vi "Pointer Convert TDMS V3.vi"() -> ()   [LabVIEW 2014]
doc: "Reads a TDMS (Technical Data Management Streaming) file."
panel:
  in  "Tab Control":enum32{"Control", "Help"}(tab)
  in  "Input path:":path
  out "Output path:":path
  out "Number of converted files:":i32
  out "Version":string
  out "array of strings":string[](array[string])
  out "channel names":string[](array[string])
  out "error out":errorcluster
  in  "error in (no error) 3":errorcluster
  in  "error in (no error) 2":errorcluster
  out "channel names 2":string[](array[string])
  out "array of strings 2":string[](array[string])
  # "Please select the folder or file you want to convert here:"
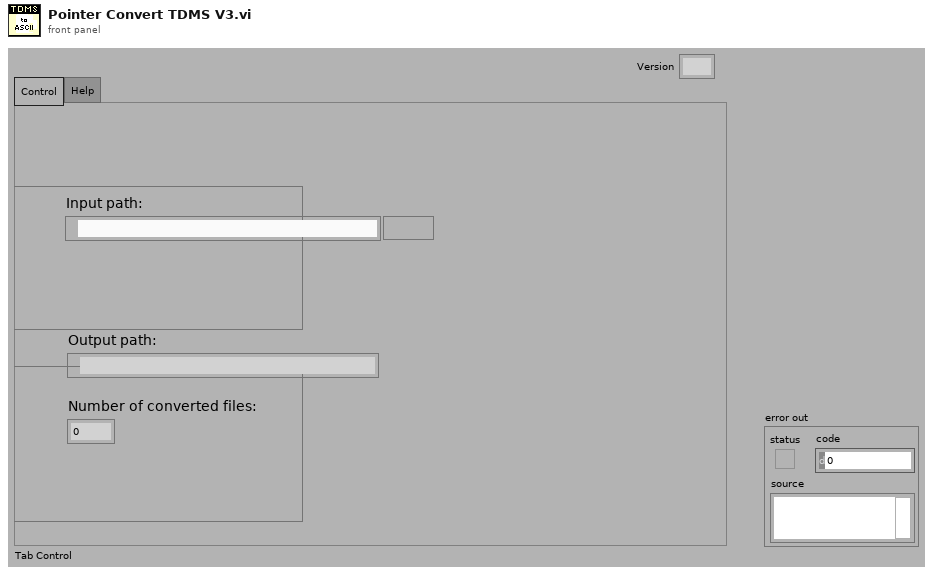
[diagram p1: front panel]
types:
  T1 = enum16{"open", "replace", "create", "open or create", "replace or create", "replace or create with confirmation"}
  T2 = enum16{"open", "open or create", "create or replace", "create", "open (read-only)"}
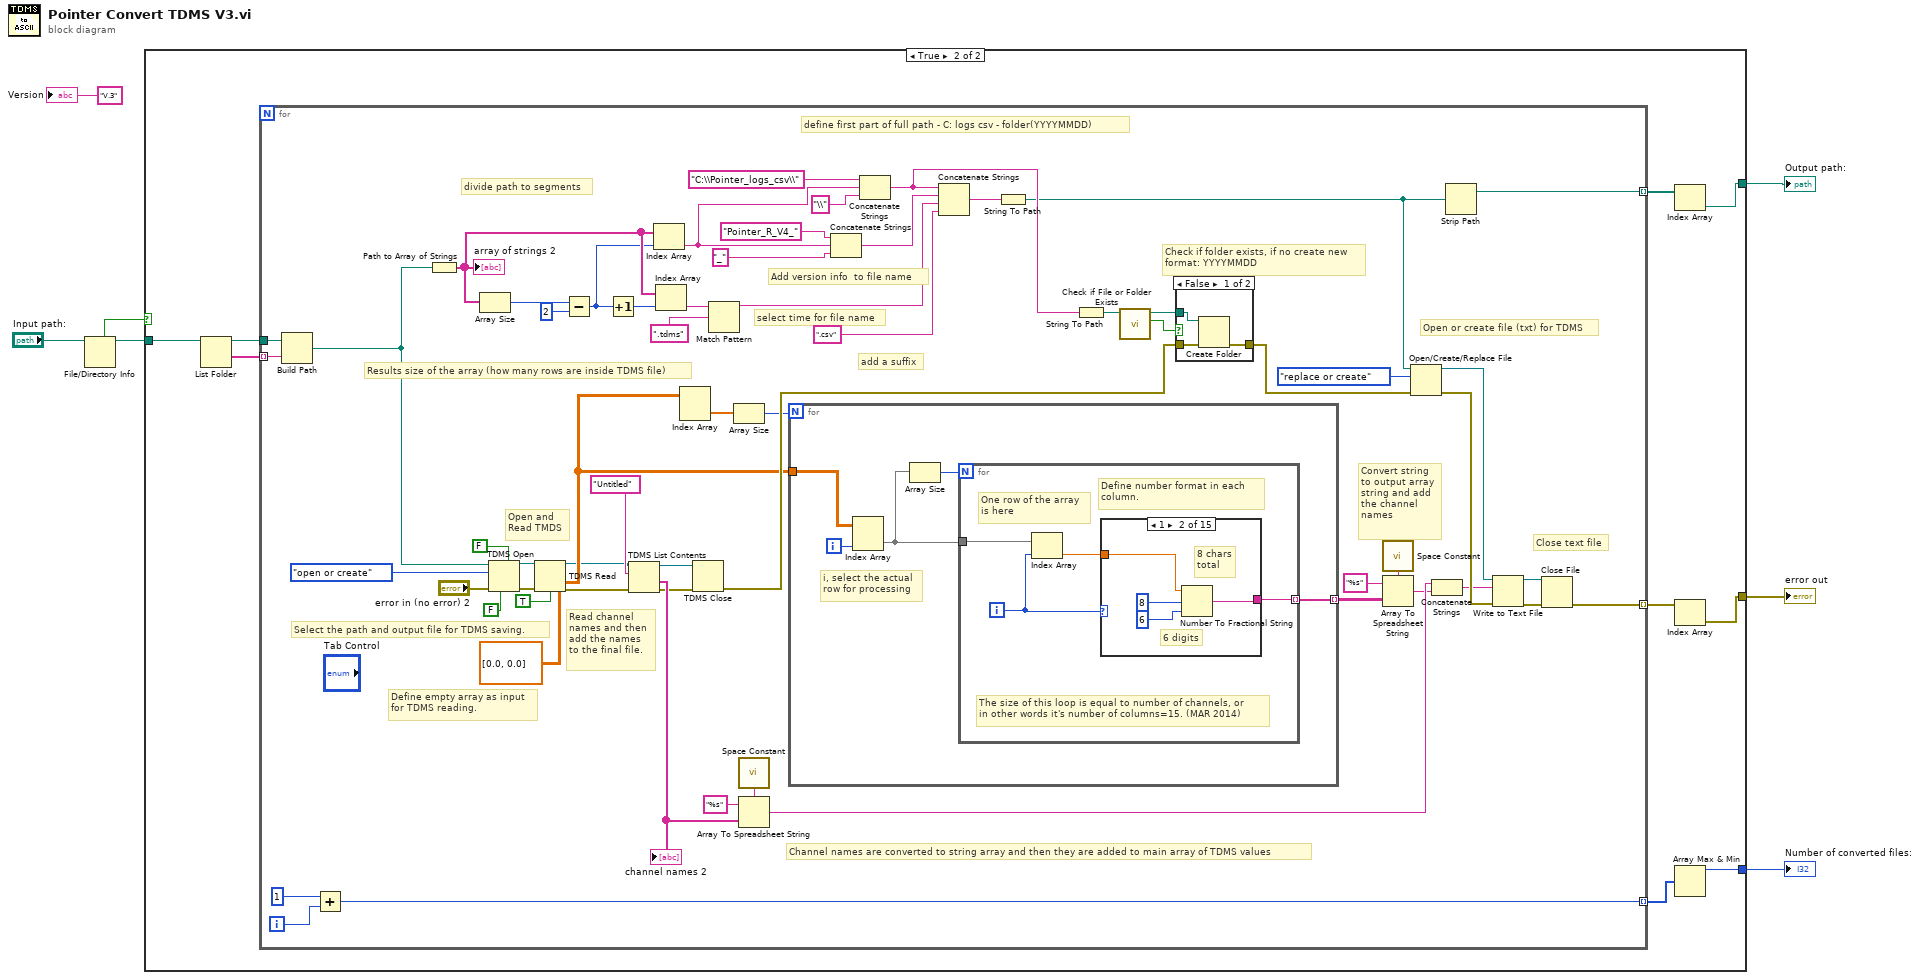
[diagram p0: block diagram]
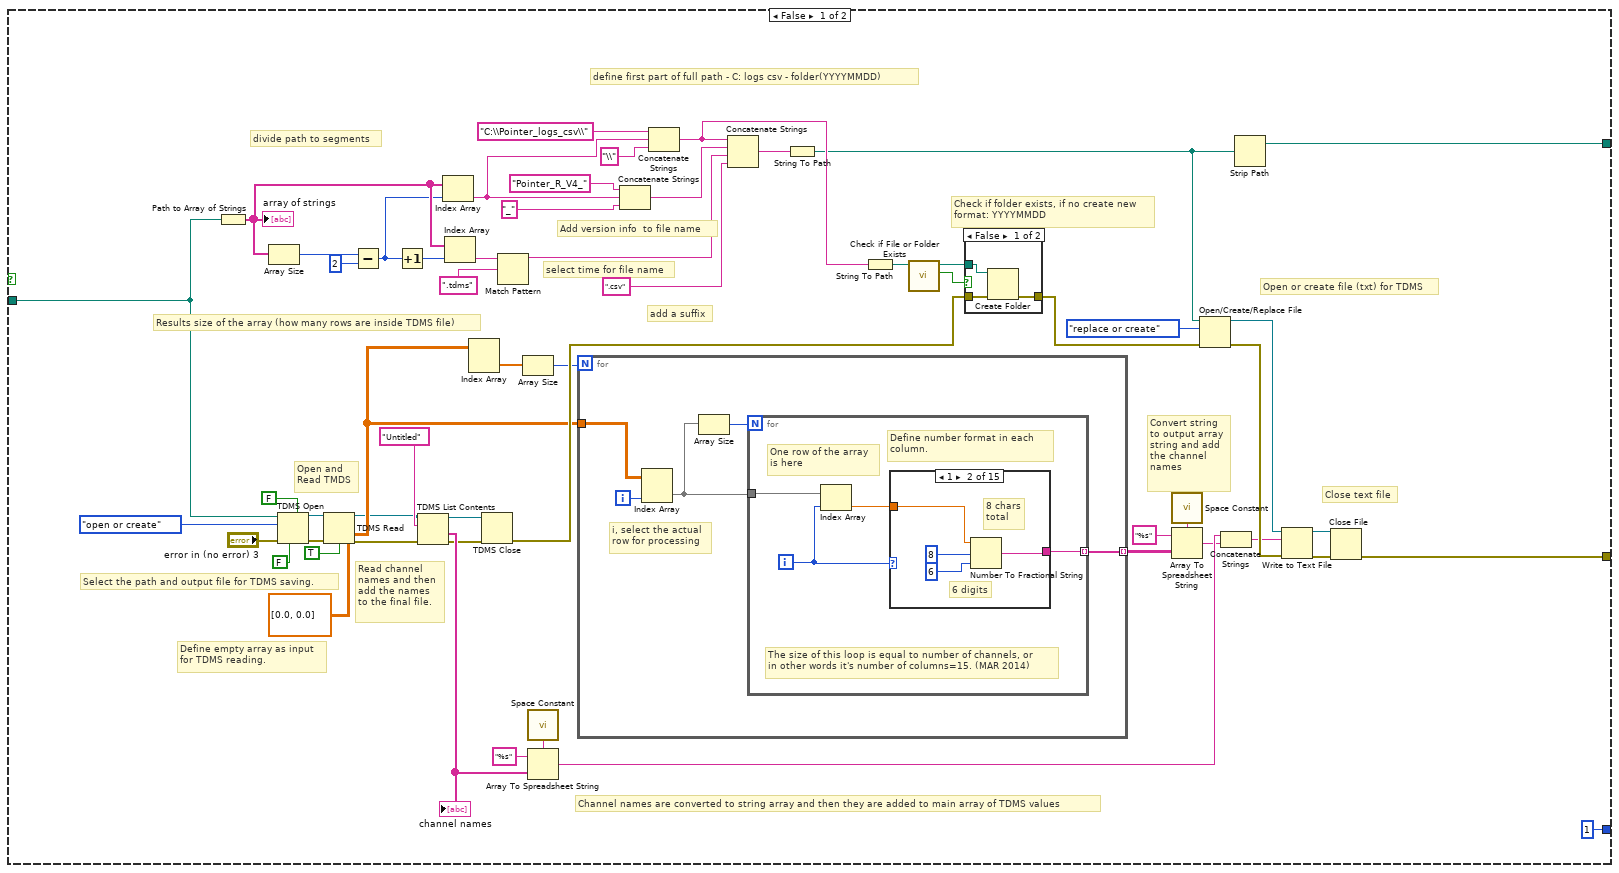
[diagram p2: hidden frame]
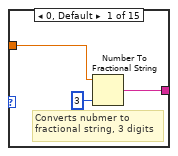
[diagram p4: hidden frame]
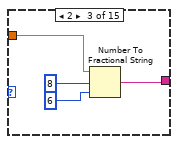
[diagram p5: hidden frame]
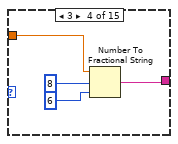
[diagram p6: hidden frame]
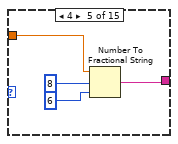
[diagram p7: hidden frame]
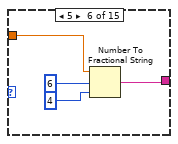
[diagram p8: hidden frame]
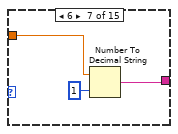
[diagram p9: hidden frame]
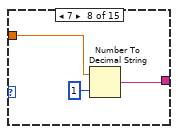
[diagram p10: hidden frame]
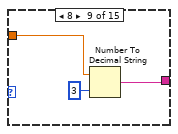
[diagram p11: hidden frame]
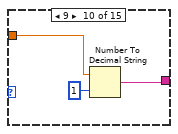
[diagram p12: hidden frame]
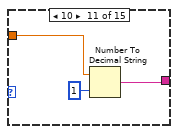
[diagram p13: hidden frame]
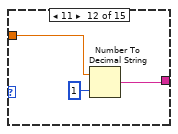
[diagram p14: hidden frame]
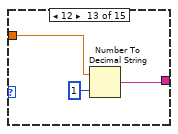
[diagram p15: hidden frame]
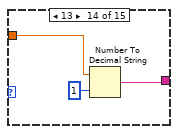
[diagram p16: hidden frame]
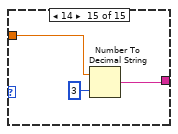
[diagram p17: hidden frame]
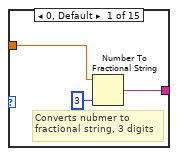
[diagram p19: hidden frame]
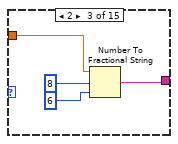
[diagram p20: hidden frame]
diagram:
  n1 = File/Directory Info(path="Input path:") -> (path out=w5:path, directory=w6:bool)  [unwired: 1 in, 5 out]
  n2 = case shown="True" w6 {
    tunnel: w5 -> [w11 w134]
    tunnel: [w10 w132] -> w4
    tunnel: [w9 w130] -> w3
    tunnel: [1 w128] -> w2
    frame False {
      # "add a suffix"
      # "select time for file name"
      # "Add version info  to file name"
      # "Check if folder exists, if no create new\nformat: YYYYMMDD"
      # "define first part of full path - C: logs csv - folder(YYYYMMDD)"
      # "divide path to segments"
      # "Open or create file (txt) for TDMS"
      # "Convert string\nto output array\nstring and add \nthe channel \nnames"
      # "Close text file"
      # "Channel names are converted to string array and then they are added to main array of TDMS values"
      # "Define empty array as input\nfor TDMS reading."
      # "Results size of the array (how many rows are inside TDMS file)"
      # "Open and \nRead TMDS"
      # "Read channel\nnames and then\nadd the names \nto the final file."
      # "Select the path and output file for TDMS saving."
      n3 = Path to Array of Strings(0:w11) -> (2:w45:string[])  [unwired: 1 out]
      "array of strings" <- w45
      n4 = Array Size(array=w45) -> (size(s)=w41:i32)
      n5 = TDMS Open(5:FALSE ("create index file? (T)"), 6:FALSE ("disable buffering (T)"), 8:"error in (no error) 3", 10:T2."open or create" ("operation"), 11:w11) -> (0:w15:errorcluster, 3:w14:refnum<k34>)  [unwired: 2 in]
      n6 = TDMS Read(0:w14, 11:w15, 12:dbl[][] [[0.0, 0.0]], 13:TRUE ("return channels in file order? (F)")) -> (4:w20:refnum<k34>, 10:w29:dbl[][], 15:w23:errorcluster)  [unwired: 4 in, 3 out]
      n7 = Subtract(x=w41, y=2) -> (x-y=w43:i32)
      n8 = Increment(x=w43) -> (x+1=w44:i32)
      n9 = TDMS List Contents(4:w23, 6:"Untitled" ("group name"), 7:w20) -> (0:w24:errorcluster, 1:w32:string[], 3:w21:refnum<k34>)  [unwired: 1 out]
      "channel names" <- w32
      n10 = Index Array(array=w45, index=w43) -> (element=w56:string)
      n11 = Index Array(array=w45, index=w44) -> (element=w47:string)
      n12 = Index Array(array=w29) -> (element=w27:dbl[])  [unwired: 2 in]
      n13 = TDMS Close(8:w24, 11:w21) -> (0:w57:errorcluster)  [unwired: 1 out]
      n14 = Match Pattern(string=w47, regular expression=".tdms") -> (before substring=w51:string)  [unwired: 1 in, 3 out]
      n15 = Array Size(array=w27) -> (size(s)=w28:i32)
      n16 = call <vilib>:"Space Constant.vi"() -> ("String"=w33:string)
      n17 = Array To Spreadsheet String(delimiter (Tab)=w33, array=w32, 3:"%s" ("format string")) -> (spreadsheet string=w37:string)
      n18 = for {
        N: w28 -> [_]
        tunnel: w29 -> [w73]
        tunnel: [w69] -> w35 mode=indexing
        i -> [w70]
        # "i, select the actual\nrow for processing"
        n19 = Index Array(array=w73, index (col)=w70) -> (element=w72:dbl[])  [unwired: 1 in]
        n20 = Array Size(array=w72) -> (size(s)=w71:i32)
        n21 = for {
          N: w71 -> [_]
          tunnel: w72 -> [w77]
          tunnel: [w75] -> w69 mode=indexing
          i -> [w74]
          # "One row of the array\nis here"
          # "Define number format in each \ncolumn."
          # "The size of this loop is equal to number of channels, or\nin other words it's number of columns=15. (MAR 2014)"
          n22 = Index Array(array=w77, index=w74) -> (element=w76:dbl)
          n23 = case shown="1" w74 {
            tunnel: w76 -> [w80 w82 w86 w90 w94 w98 w102 w105 w108 w111 w114 w117 w120 w123 w126]
            tunnel: [w79 w83 w87 w91 w95 w99 w103 w106 w109 w112 w115 w118 w121 w124 w127] -> w75
            frame 0, Default {
              # "Converts nubmer to \nfractional string, 3 digits"
              n24 = Number To Fractional String(number=w80, precision (6)=i16 3) -> (F-format string=w79:string)  [unwired: 2 in]
            }
            frame 1 {
              # "6 digits"
              # "8 chars\ntotal"
              n25 = Number To Fractional String(number=w82, width (-)=i16 8, precision (6)=i16 6) -> (F-format string=w83:string)  [unwired: 1 in]
            }
            frame 2 {
              n26 = Number To Fractional String(number=w86, width (-)=i16 8, precision (6)=i16 6) -> (F-format string=w87:string)  [unwired: 1 in]
            }
            frame 3 {
              n27 = Number To Fractional String(number=w90, width (-)=i16 8, precision (6)=i16 6) -> (F-format string=w91:string)  [unwired: 1 in]
            }
            frame 4 {
              n28 = Number To Fractional String(number=w94, width (-)=i16 8, precision (6)=i16 6) -> (F-format string=w95:string)  [unwired: 1 in]
            }
            frame 5 {
              n29 = Number To Fractional String(number=w98, width (-)=i16 6, precision (6)=i16 4) -> (F-format string=w99:string)  [unwired: 1 in]
            }
            frame 6 {
              n30 = Number To Decimal String(number=w102, width (-)=i16 1) -> (decimal integer string=w103:string)
            }
            frame 7 {
              n31 = Number To Decimal String(number=w105, width (-)=i16 1) -> (decimal integer string=w106:string)
            }
            frame 8 {
              n32 = Number To Decimal String(number=w108, width (-)=i16 3) -> (decimal integer string=w109:string)
            }
            frame 9 {
              n33 = Number To Decimal String(number=w111, width (-)=i16 1) -> (decimal integer string=w112:string)
            }
            frame 10 {
              n34 = Number To Decimal String(number=w114, width (-)=i16 1) -> (decimal integer string=w115:string)
            }
            frame 11 {
              n35 = Number To Decimal String(number=w117, width (-)=i16 1) -> (decimal integer string=w118:string)
            }
            frame 12 {
              n36 = Number To Decimal String(number=w120, width (-)=i16 1) -> (decimal integer string=w121:string)
            }
            frame 13 {
              n37 = Number To Decimal String(number=w123, width (-)=i16 1) -> (decimal integer string=w124:string)
            }
            frame 14 {
              n38 = Number To Decimal String(number=w126, width (-)=i16 3) -> (decimal integer string=w127:string)
            }
          }
        }
      }
      n39 = Concatenate Strings("Pointer_R_V4_" ("string"), w56, "_" ("string")) -> (w50:string)
      n40 = Concatenate Strings("C:\\Pointer_logs_csv\\", w56, "\\") -> (w59:string)
      n41 = Concatenate Strings(w59, w50, w51, ".csv" ("string")) -> (w52:string)
      n42 = String To Path(string=w52) -> (path=w12:path)
      n43 = String To Path(string=w59) -> (path=w60:path)
      n44 = call <vilib>:"Check if File or Folder Exists.vi"("path"=w60) -> ("file or folder exists?"=w61:bool, "dup path"=w62:path)  [unwired: 8 in, 1 out]
      n45 = case shown="False" w61 {
        tunnel: w57 -> [w67 w68]
        tunnel: [w66 w68] -> w58
        tunnel: w62 -> [w65 _]
        frame False {
          n46 = Create Folder(path (use dialog)=w65, error in=w67) -> (error out=w66:errorcluster)  [unwired: 1 in, 2 out]
        }
        frame True {
        }
      }
      n47 = call <vilib>:"Space Constant.vi"() -> ("String"=w31:string)
      n48 = Array To Spreadsheet String(delimiter (Tab)=w31, array=w35, 3:"%s" ("format string")) -> (spreadsheet string=w36:string)
      n49 = Open/Create/Replace File(file path (use dialog)=w12, error in=w58, operation (0:open)=T1."replace or create") -> (refnum out=w39:refnum<file>, error out=w40:errorcluster)  [unwired: 3 in, 1 out]
      n50 = Concatenate Strings(w37, w36) -> (w38:string)
      n51 = Strip Path(path=w12) -> (stripped path=w10:path)  [unwired: 1 out]
      n52 = Write to Text File(file (use dialog)=w39, text=w38, error in=w40) -> (refnum out=w25:refnum<file>, error out=w26:errorcluster)  [unwired: 1 in, 1 out]
      n53 = Close File(refnum=w25, error in=w26) -> (error out=w9:errorcluster)  [unwired: 1 out]
    }
    frame True {
      n54 = List Folder(path=w134) -> (path out=w135:path, filenames=w136:string[])  [unwired: 3 in, 2 out]
      n55 = for {
        tunnel: w136 -> [w196] mode=indexing
        tunnel: w135 -> [w197]
        tunnel: [w141] -> w133 mode=indexing
        tunnel: [w140] -> w131 mode=indexing
        tunnel: [w137] -> w129 mode=indexing
        i -> [w139]
        # "add a suffix"
        # "select time for file name"
        # "Add version info  to file name"
        # "Check if folder exists, if no create new\nformat: YYYYMMDD"
        # "define first part of full path - C: logs csv - folder(YYYYMMDD)"
        # "divide path to segments"
        # "Open or create file (txt) for TDMS"
        # "Convert string\nto output array\nstring and add \nthe channel \nnames"
        # "Close text file"
        # "Channel names are converted to string array and then they are added to main array of TDMS values"
        # "Define empty array as input\nfor TDMS reading."
        # "Results size of the array (how many rows are inside TDMS file)"
        # "Open and \nRead TMDS"
        # "Read channel\nnames and then\nadd the names \nto the final file."
        # "Select the path and output file for TDMS saving."
        n56 = Build Path(base path=w197, name or relative path=w196) -> (appended path=w143:path)
        n57 = Add(x=1, y=w139) -> (x+y=w137:i32)
        n58 = Path to Array of Strings(0:w143) -> (2:w176:string[])  [unwired: 1 out]
        "array of strings 2" <- w176
        n59 = Array Size(array=w176) -> (size(s)=w172:i32)
        n60 = TDMS Open(5:FALSE ("create index file? (T)"), 6:FALSE ("disable buffering (T)"), 8:"error in (no error) 2", 10:T2."open or create" ("operation"), 11:w143) -> (0:w146:errorcluster, 3:w145:refnum<k34>)  [unwired: 2 in]
        n61 = TDMS Read(0:w145, 11:w146, 12:dbl[][] [[0.0, 0.0]], 13:TRUE ("return channels in file order? (F)")) -> (4:w151:refnum<k34>, 10:w160:dbl[][], 15:w154:errorcluster)  [unwired: 4 in, 3 out]
        n62 = Subtract(x=w172, y=2) -> (x-y=w174:i32)
        n63 = Increment(x=w174) -> (x+1=w175:i32)
        n64 = TDMS List Contents(4:w154, 6:"Untitled" ("group name"), 7:w151) -> (0:w155:errorcluster, 1:w163:string[], 3:w152:refnum<k34>)  [unwired: 1 out]
        "channel names 2" <- w163
        n65 = Index Array(array=w176, index=w174) -> (element=w187:string)
        n66 = Index Array(array=w176, index=w175) -> (element=w178:string)
        n67 = Index Array(array=w160) -> (element=w158:dbl[])  [unwired: 2 in]
        n68 = TDMS Close(8:w155, 11:w152) -> (0:w188:errorcluster)  [unwired: 1 out]
        n69 = Match Pattern(string=w178, regular expression=".tdms") -> (before substring=w182:string)  [unwired: 1 in, 3 out]
        n70 = Array Size(array=w158) -> (size(s)=w159:i32)
        n71 = call <vilib>:"Space Constant.vi"() -> ("String"=w164:string)
        n72 = Array To Spreadsheet String(delimiter (Tab)=w164, array=w163, 3:"%s" ("format string")) -> (spreadsheet string=w168:string)
        n73 = for {
          N: w159 -> [_]
          tunnel: w160 -> [w206]
          tunnel: [w202] -> w166 mode=indexing
          i -> [w203]
          # "i, select the actual\nrow for processing"
          n74 = Index Array(array=w206, index (col)=w203) -> (element=w205:dbl[])  [unwired: 1 in]
          n75 = Array Size(array=w205) -> (size(s)=w204:i32)
          n76 = for {
            N: w204 -> [_]
            tunnel: w205 -> [w210]
            tunnel: [w208] -> w202 mode=indexing
            i -> [w207]
            # "One row of the array\nis here"
            # "Define number format in each \ncolumn."
            # "The size of this loop is equal to number of channels, or\nin other words it's number of columns=15. (MAR 2014)"
            n77 = Index Array(array=w210, index=w207) -> (element=w209:dbl)
            n78 = case shown="1" w207 {
              tunnel: w209 -> [w213 w215 w219 w223 w227 w231 w235 w238 w241 w244 w247 w250 w253 w256 w259]
              tunnel: [w212 w216 w220 w224 w228 w232 w236 w239 w242 w245 w248 w251 w254 w257 w260] -> w208
              frame 0, Default {
                # "Converts nubmer to \nfractional string, 3 digits"
                n79 = Number To Fractional String(number=w213, precision (6)=i16 3) -> (F-format string=w212:string)  [unwired: 2 in]
              }
              frame 1 {
                # "6 digits"
                # "8 chars\ntotal"
                n80 = Number To Fractional String(number=w215, width (-)=i16 8, precision (6)=i16 6) -> (F-format string=w216:string)  [unwired: 1 in]
              }
              frame 2 {
                n81 = Number To Fractional String(number=w219, width (-)=i16 8, precision (6)=i16 6) -> (F-format string=w220:string)  [unwired: 1 in]
              }
              frame 3 {
                n82 = Number To Fractional String(number=w223, width (-)=i16 8, precision (6)=i16 6) -> (F-format string=w224:string)  [unwired: 1 in]
              }
              frame 4 {
                n83 = Number To Fractional String(number=w227, width (-)=i16 8, precision (6)=i16 6) -> (F-format string=w228:string)  [unwired: 1 in]
              }
              frame 5 {
                n84 = Number To Fractional String(number=w231, width (-)=i16 6, precision (6)=i16 4) -> (F-format string=w232:string)  [unwired: 1 in]
              }
              frame 6 {
                n85 = Number To Decimal String(number=w235, width (-)=i16 1) -> (decimal integer string=w236:string)
              }
              frame 7 {
                n86 = Number To Decimal String(number=w238, width (-)=i16 1) -> (decimal integer string=w239:string)
              }
              frame 8 {
                n87 = Number To Decimal String(number=w241, width (-)=i16 3) -> (decimal integer string=w242:string)
              }
              frame 9 {
                n88 = Number To Decimal String(number=w244, width (-)=i16 1) -> (decimal integer string=w245:string)
              }
              frame 10 {
                n89 = Number To Decimal String(number=w247, width (-)=i16 1) -> (decimal integer string=w248:string)
              }
              frame 11 {
                n90 = Number To Decimal String(number=w250, width (-)=i16 1) -> (decimal integer string=w251:string)
              }
              frame 12 {
                n91 = Number To Decimal String(number=w253, width (-)=i16 1) -> (decimal integer string=w254:string)
              }
              frame 13 {
                n92 = Number To Decimal String(number=w256, width (-)=i16 1) -> (decimal integer string=w257:string)
              }
              frame 14 {
                n93 = Number To Decimal String(number=w259, width (-)=i16 3) -> (decimal integer string=w260:string)
              }
            }
          }
        }
        n94 = Concatenate Strings("Pointer_R_V4_" ("string"), w187, "_" ("string")) -> (w181:string)
        n95 = Concatenate Strings("C:\\Pointer_logs_csv\\", w187, "\\") -> (w190:string)
        n96 = Concatenate Strings(w190, w181, w182, ".csv" ("string")) -> (w183:string)
        n97 = String To Path(string=w183) -> (path=w142:path)
        n98 = String To Path(string=w190) -> (path=w191:path)
        n99 = call <vilib>:"Check if File or Folder Exists.vi"("path"=w191) -> ("file or folder exists?"=w192:bool, "dup path"=w193:path)  [unwired: 8 in, 1 out]
        n100 = case shown="False" w192 {
          tunnel: w188 -> [w200 w201]
          tunnel: [w199 w201] -> w189
          tunnel: w193 -> [w198 _]
          frame False {
            n101 = Create Folder(path (use dialog)=w198, error in=w200) -> (error out=w199:errorcluster)  [unwired: 1 in, 2 out]
          }
          frame True {
          }
        }
        n102 = call <vilib>:"Space Constant.vi"() -> ("String"=w162:string)
        n103 = Array To Spreadsheet String(delimiter (Tab)=w162, array=w166, 3:"%s" ("format string")) -> (spreadsheet string=w167:string)
        n104 = Open/Create/Replace File(file path (use dialog)=w142, error in=w189, operation (0:open)=T1."replace or create") -> (refnum out=w170:refnum<file>, error out=w171:errorcluster)  [unwired: 3 in, 1 out]
        n105 = Concatenate Strings(w168, w167) -> (w169:string)
        n106 = Strip Path(path=w142) -> (stripped path=w141:path)  [unwired: 1 out]
        n107 = Write to Text File(file (use dialog)=w170, text=w169, error in=w171) -> (refnum out=w156:refnum<file>, error out=w157:errorcluster)  [unwired: 1 in, 1 out]
        n108 = Close File(refnum=w156, error in=w157) -> (error out=w140:errorcluster)  [unwired: 1 out]
      }
      n109 = Index Array(array=w133) -> (element=w132:path)  [unwired: 1 in]
      n110 = Index Array(array=w131) -> (element=w130:errorcluster)  [unwired: 1 in]
      n111 = Array Max & Min(array=w129) -> (max value=w128:i32)  [unwired: 3 out]
    }
  }
  "Output path:" <- w4
  "error out" <- w3
  "Number of converted files:" <- w2
  "Version" <- "V.3" ("Version")
